vi "Generate simulated control timings sequence.vi"(7 "ROI Dwell time":dbl, 9 "High value of simulated waveform":dbl, 10 "Time resolution of simulated waveform":dbl, 11 "Number of POI":i32) -> (3 "Simulated control timings sequence in":waveform(dbl))   [LabVIEW 2013]
uses:
  Global Variables/General Globals.vi
  <vilib>/Waveform/WDTOps.llb/WDT Append Waveforms DBL.vi
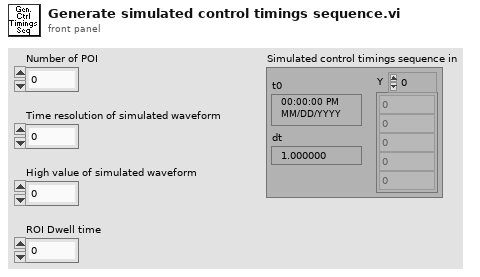
[diagram p1: front panel]
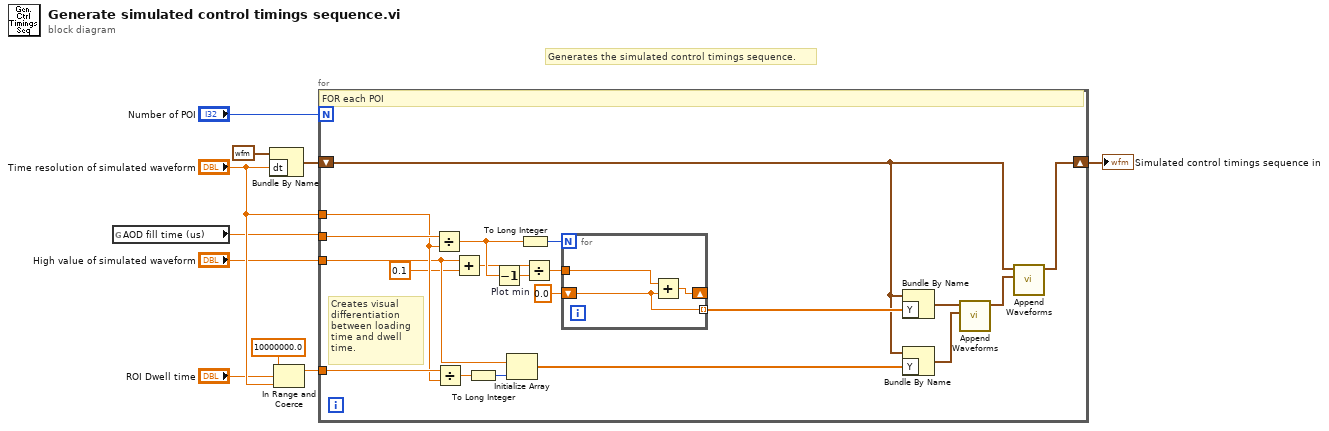
[diagram p0: block diagram]
diagram:
  # "Generates the simulated control timings sequence."
  n1 = global read "General Globals.vi" "AOD fill time (us)"() -> (w6:dbl)
  n2 = Bundle By Name ("Build Waveform")(cluster=waveform(dbl) {"t0"=timestamp(0 s since 1904-01-01), "dt"=0.0, "Y"=[]} ("waveform out"), "dt"="Time resolution of simulated waveform") -> (w1:waveform(dbl))
  n3 = In Range and Coerce(upper limit=10000000.0, x="ROI Dwell time", lower limit="Time resolution of simulated waveform") -> (coerced(x)=w4:dbl)  [unwired: 1 out]
  n4 = for {
    N: "Number of POI" -> [_]
    shift-right: [w23] -> w7
    shift-left: w1 -> [w14]
    tunnel: "Time resolution of simulated waveform" -> [w15]
    tunnel: w4 -> [w18]
    tunnel: w6 -> [w17]
    tunnel: "High value of simulated waveform" -> [w13]
    w30 = 0.0  # Plot min
    # "Creates visual differentiation between loading time and dwell time."
    # "FOR each POI"
    n5 = Divide(x=w17, y=w15) -> (x/y=w20:dbl)
    n6 = Divide(x=w18, y=w15) -> (x/y=w28:dbl)
    n7 = Add(x=w13, y=0.1) -> (x+y=w12:dbl)
    n8 = To Long Integer(number=w28) -> (32bit integer=w27:i32)
    n9 = Decrement(x=w20) -> (x-1=w19:dbl)
    n10 = Initialize Array(w13, w27) -> (w26:dbl[])
    n11 = To Long Integer(number=w20) -> (32bit integer=w21:i32)
    n12 = Divide(x=w12, y=w19) -> (x/y=w29:dbl)
    n13 = for {
      N: w21 -> [_]
      shift-right: [w32] -> _
      shift-left: w30 -> [w31]
      tunnel: w29 -> [w33]
      tunnel: [w31] -> w16 mode=indexing
      n14 = Add(x=w33, y=w31) -> (x+y=w32:dbl)
    }
    n15 = Bundle By Name(cluster=w14, "Y"=w16) -> (w25:waveform(dbl))
    n16 = Bundle By Name(cluster=w14, "Y"=w26) -> (w24:waveform(dbl))
    n17 = call-poly <vilib>:"Append Waveforms.vi"("waveform B"=w24, "waveform A"=w25) -> ("waveform out"=w22:waveform(dbl))  [unwired: 8 in, 1 out]
    n18 = call-poly <vilib>:"Append Waveforms.vi"("waveform B"=w22, "waveform A"=w14) -> ("waveform out"=w23:waveform(dbl))  [unwired: 8 in, 1 out]
  }
  "Simulated control timings sequence in" <- w7
